vi "TAT_Varient Creater.vi"(8 "error in (no error)":errorcluster) -> (0 "error out":errorcluster)   [LabVIEW 2017]
uses:
  <vilib>/Utility/config.llb/Read Key (I32).vi
  <vilib>/Utility/config.llb/Write Key (U32).vi
  <vilib>/Utility/config.llb/NI_LVConfig.lvlib
  557cc533-a4ba-4953-a7b5-ba01b5e60265.vi
panel:
  in  "Cancle 2":bool
  in  "Delete Button":bool
  in  "Save Button":bool
  out "Varient Details":string[][](table)
  in  "SERIAL  NUMBER":u16=1 min=1 max=100 step=1
  in  "HOME":bool
  in  "UPDATE TABLE":bool
  in  "FG CAT No.":string(combo)
  # "Varient Creater"
  # "NOT IN USE"
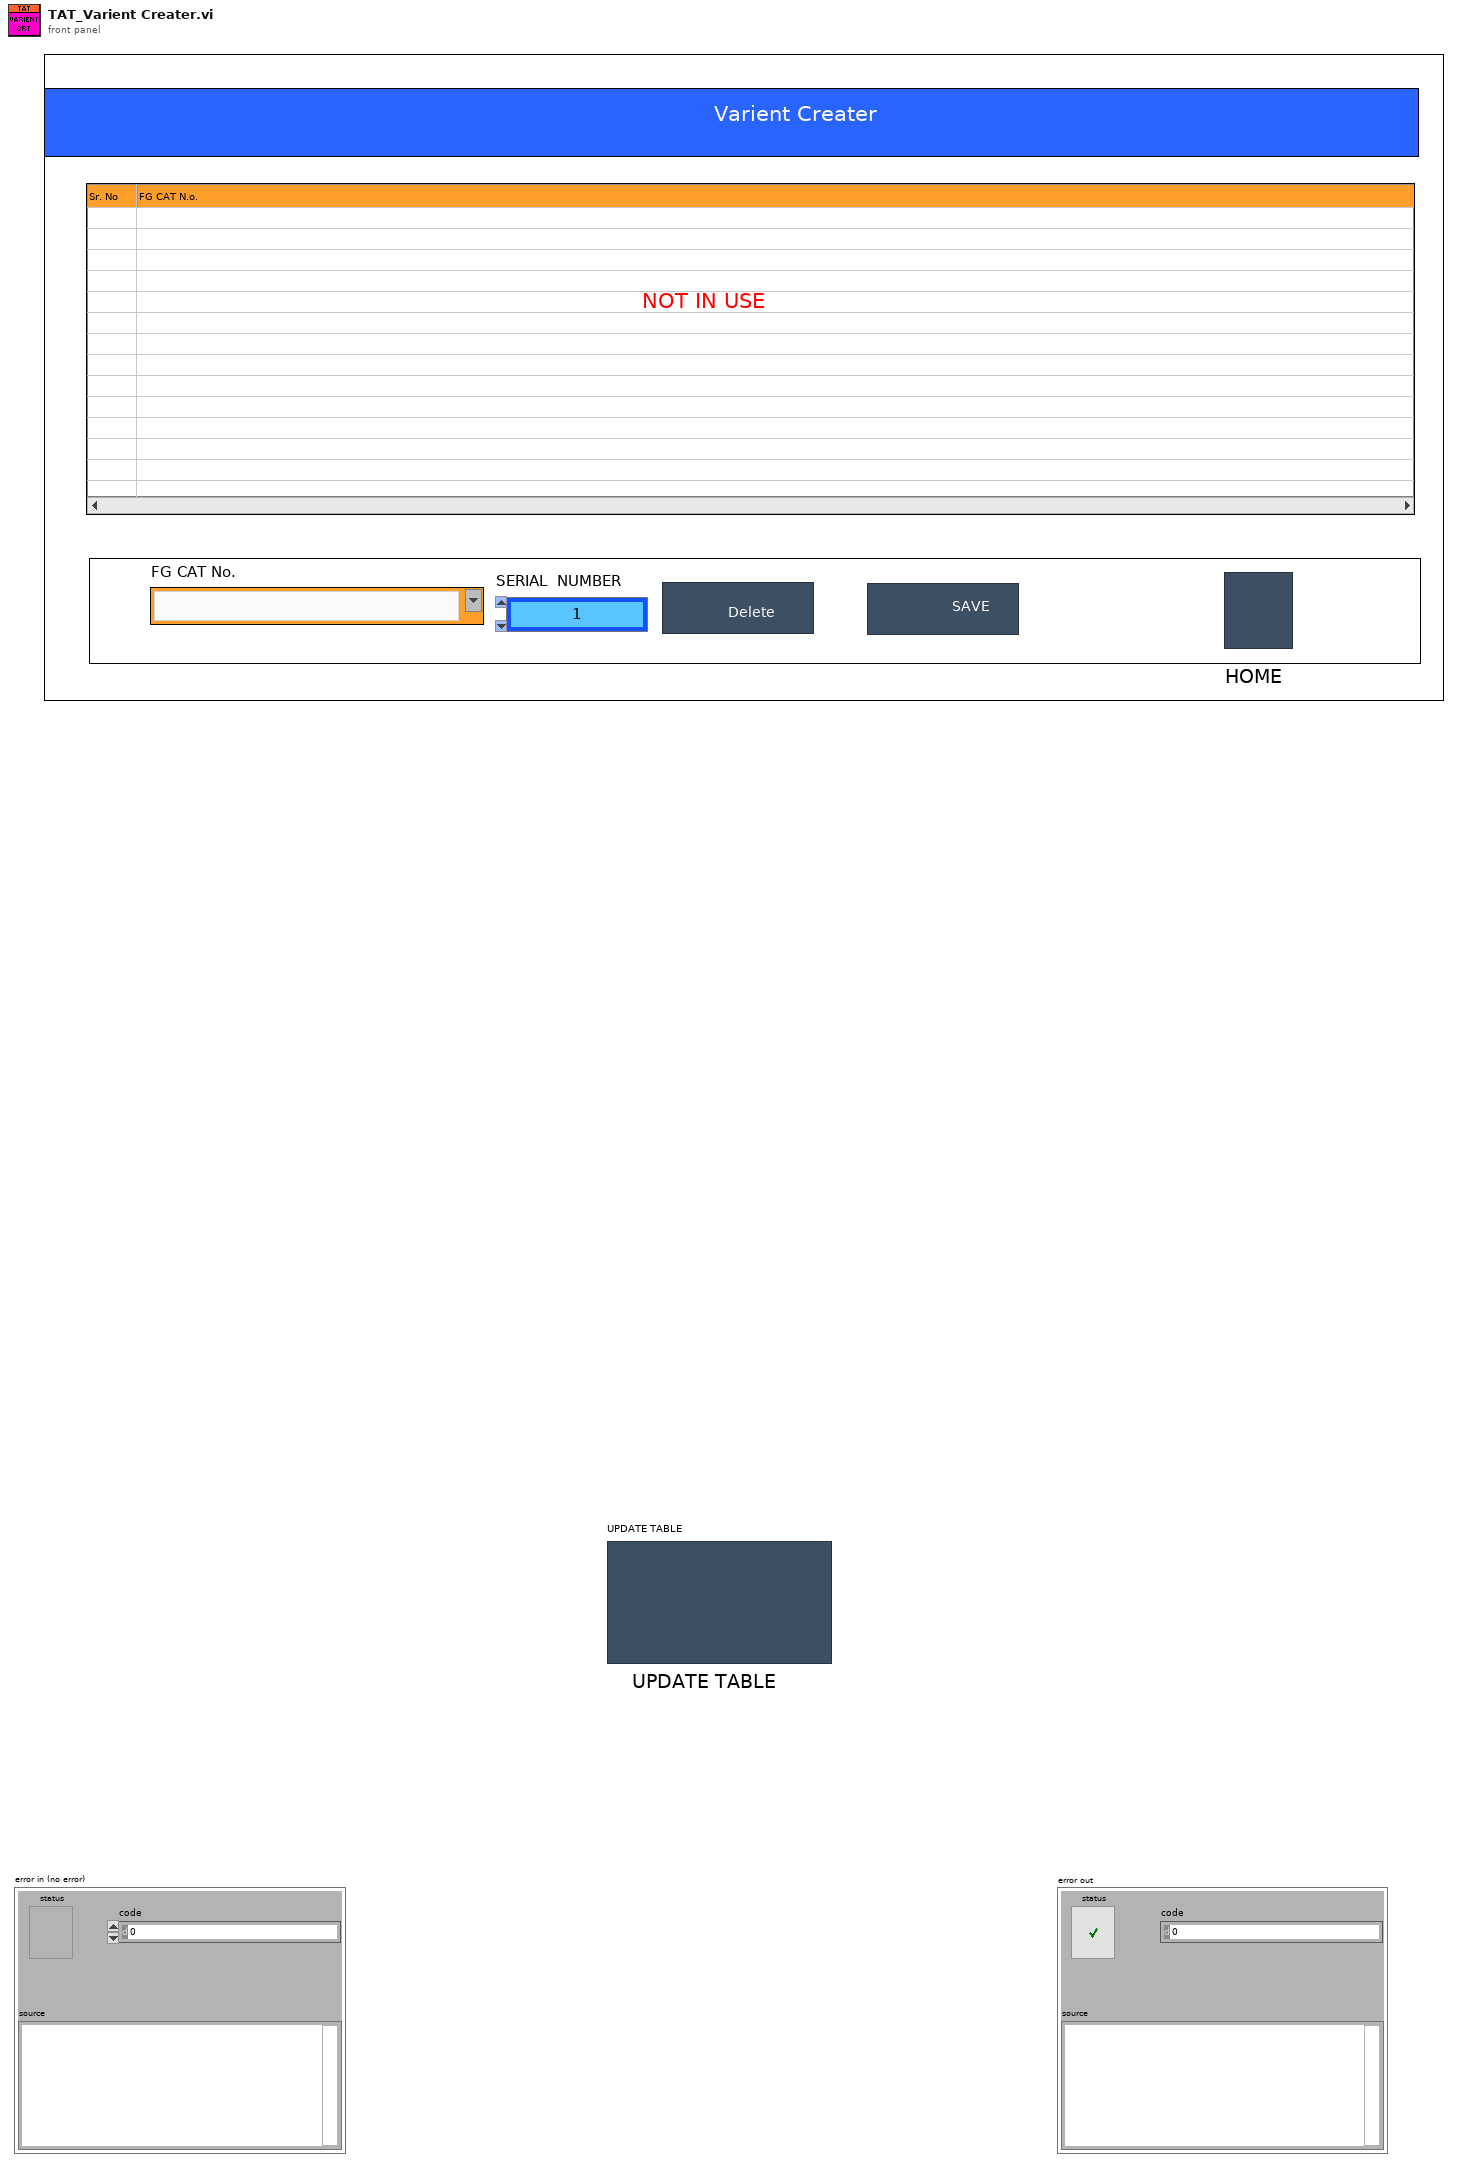
[diagram p1: front panel]
types:
  T1 = enum32{"invalid app kind", "Development System", "Run Time System", "Student Edition", "Embedded LabVIEW", "Evaluation", "Custom"}
  T2 = typedef "NI_LVConfig.lvlib/Config Data RefNum.ctl" = refnum<k1>
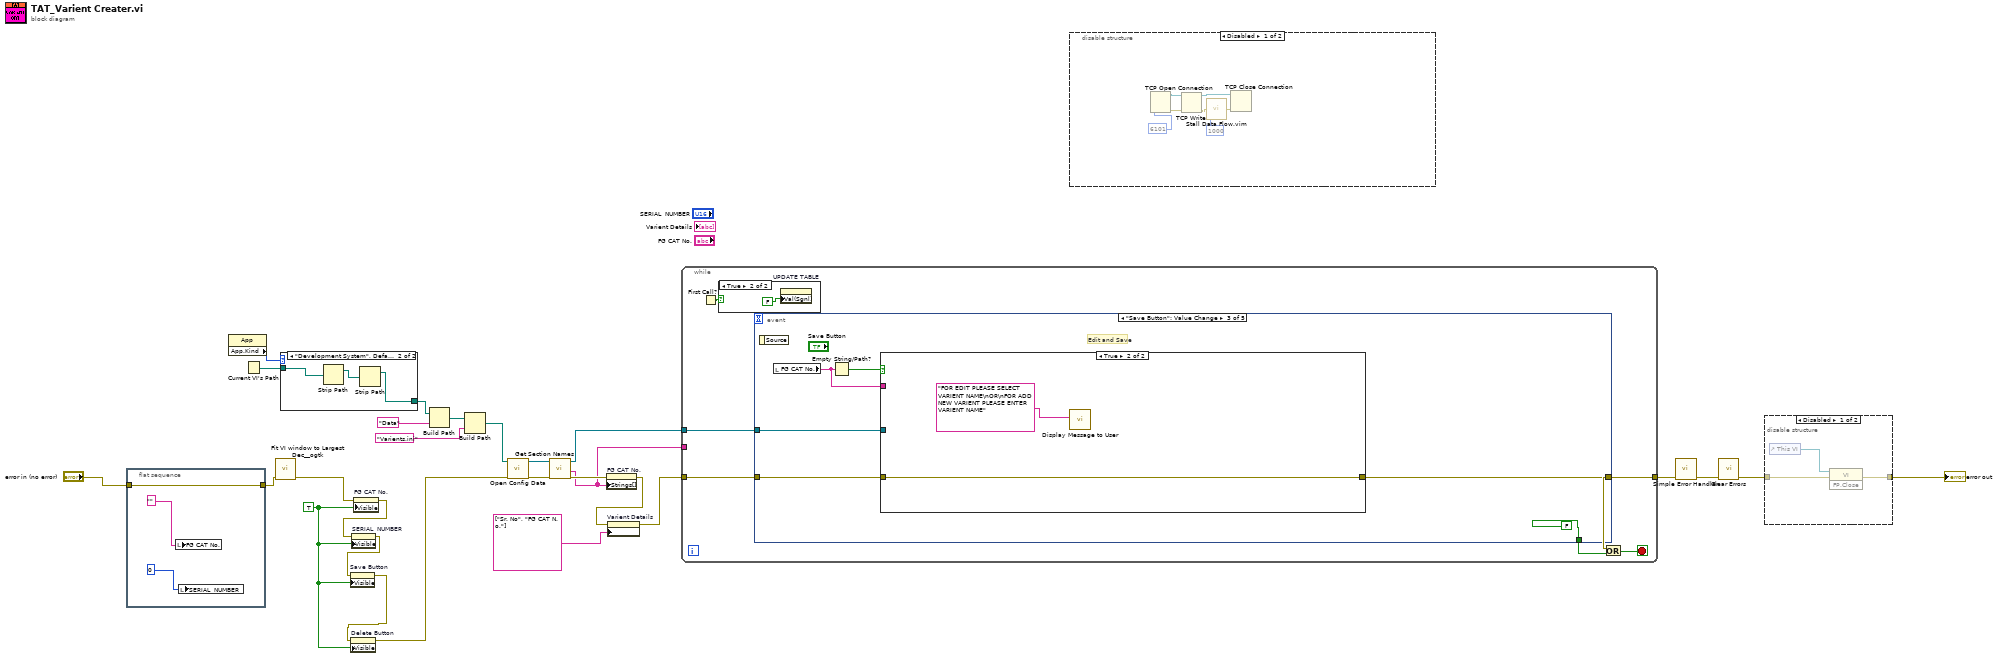
[diagram p0: block diagram]
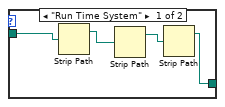
[diagram p4: hidden frame]
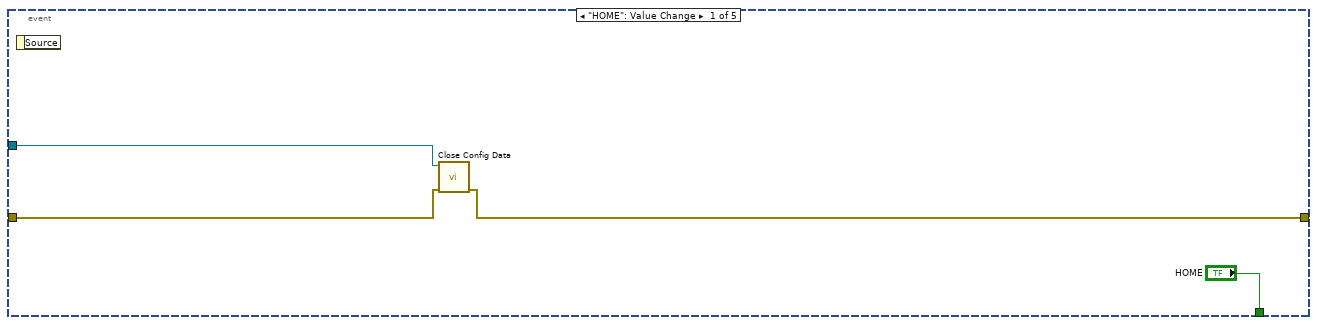
[diagram p6: hidden frame]
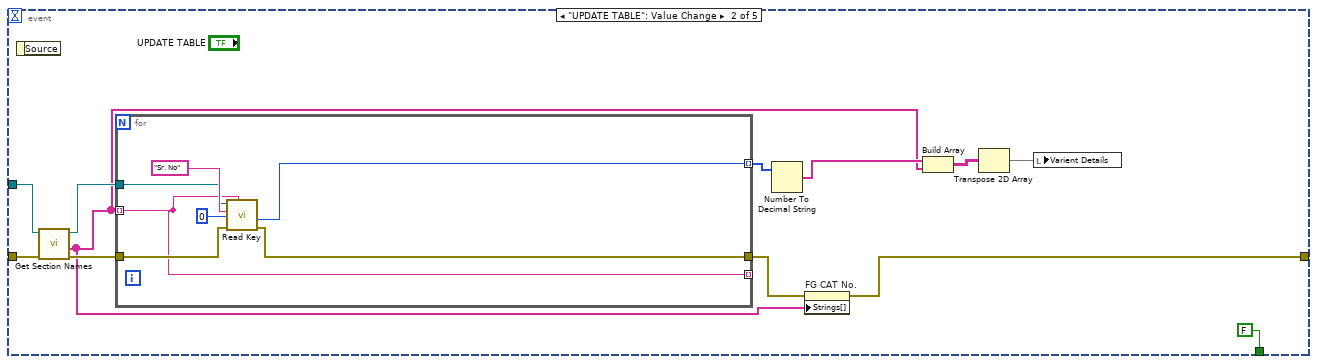
[diagram p7: hidden frame]
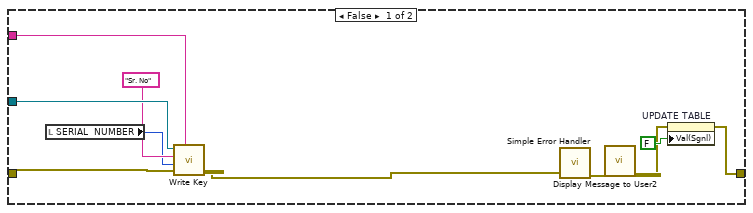
[diagram p8: hidden frame]
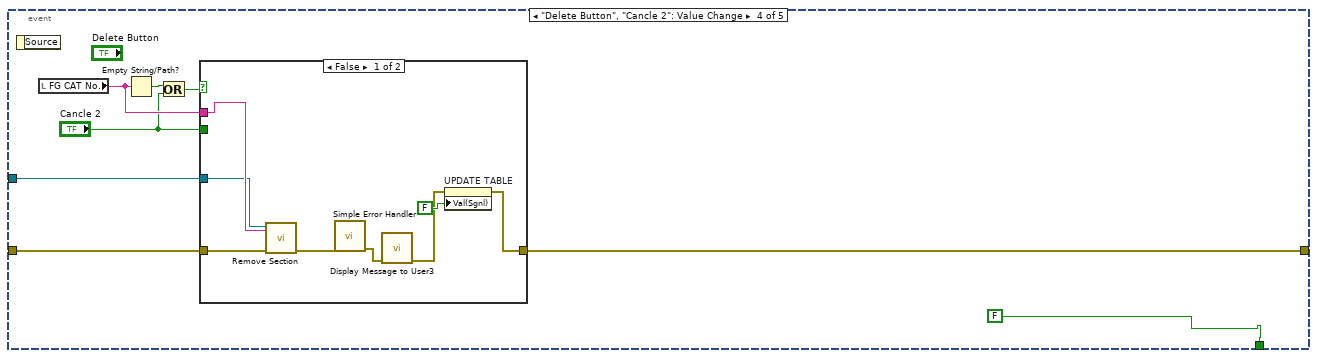
[diagram p9: hidden frame]
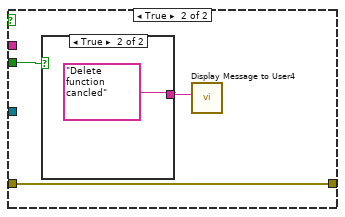
[diagram p10: hidden frame]
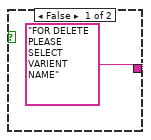
[diagram p11: hidden frame]
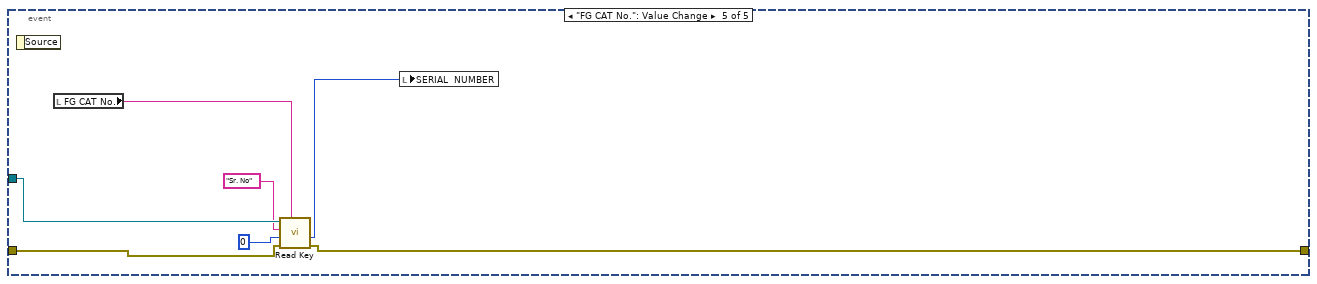
[diagram p12: hidden frame]
diagram:
  w5 = TRUE
  n1 = flat-sequence {
    tunnel: [w30] -> w10
    tunnel: "error in (no error)" -> [w30]
    frame #0 {
      n2 = local write "FG CAT No."("" ("PART NUMBER")) -> ()
      n3 = local write "SERIAL  NUMBER"(u16 0 ("BATCH SIZE")) -> ()
    }
  }
  n4 = property class="App"() -> ("App.Kind"=w22:T1)  [unwired: 2 in, 2 out]
  n5 = Current VI's Path() -> (path=w23:path)
  n6 = call <userlib>:"Fit VI window to Largest Dec__ogtk.vi"("error in (no error)"=w10) -> ("error out"=w3:errorcluster)  [unwired: 5 in, 1 out]
  n7 = case shown="\"Development System\", Default" w22 {
    tunnel: w23 -> [w32 w36]
    tunnel: [w31 w35] -> w6
    frame "Run Time System" {
      n8 = Strip Path(path=w32) -> (stripped path=w34:path)  [unwired: 1 out]
      n9 = Strip Path(path=w34) -> (stripped path=w33:path)  [unwired: 1 out]
      n10 = Strip Path(path=w33) -> (stripped path=w31:path)  [unwired: 1 out]
    }
    frame "Development System", Default {
      n11 = Strip Path(path=w36) -> (stripped path=w37:path)  [unwired: 1 out]
      n12 = Strip Path(path=w37) -> (stripped path=w35:path)  [unwired: 1 out]
    }
  }
  n13 = property on="FG CAT No." class="CmbBox"(error in=w3, "Visible"=w5) -> (error out=w9:errorcluster)  [unwired: 1 in, 1 out]
  n14 = property on="SERIAL  NUMBER" class="DigNum (strict)"(error in=w9, "Visible"=w5) -> (error out=w2:errorcluster)  [unwired: 1 in, 1 out]
  n15 = property on="Save Button" class="Bool"(error in=w2, "Visible"=w5) -> (error out=w1:errorcluster)  [unwired: 1 in, 1 out]
  n16 = property on="Delete Button" class="Bool"(error in=w1, "Visible"=w5) -> (error out=w8:errorcluster)  [unwired: 1 in, 1 out]
  n17 = Build Path(base path=w6, name or relative path="Data") -> (appended path=w7:path)
  n18 = Build Path(base path=w7, name or relative path="Varients.ini") -> (appended path=w21:path)
  n19 = call <vilib>:"Open Config Data.vi"("error in (no error)"=w8, "configuration file path"=w21) -> ("error out"=w17:errorcluster, "refnum"=w18:T2)  [unwired: 7 in, 1 out]
  n20 = call <vilib>:"Get Section Names.vi"("error in (no error)"=w17, "refnum"=w18) -> ("error out"=w16:errorcluster, "section names"=w12:string[], "refnum out"=w15:T2)  [unwired: 7 in]
  n21 = property on="FG CAT No." class="CmbBox"(error in=w16, "Strings[]"=w12) -> (error out=w14:errorcluster)  [unwired: 1 in, 1 out]
  n22 = property on="Varient Details" class="Tbl (strict)"(error in=w14, "Column Headers[]"=string[] ["Sr. No", "FG CAT N.o."]) -> (error out=w13:errorcluster)  [unwired: 1 in, 1 out]
  n23 = while {
    tunnel: w13 -> [w42]
    tunnel: [w40] -> w24
    tunnel: w15 -> [w39]
    tunnel: w12 -> [_]
    stop <- w41 stop-if-true
    n24 = First Call?() -> (First Call?: T/F=w38:bool)
    n25 = case shown="True" w38 {
      frame False {
      }
      frame True {
        n26 = property on="UPDATE TABLE" class="Bool (strict)"("Val(Sgnl)"=FALSE) -> ()  [unwired: 2 in, 2 out]
      }
    }
    n27 = event shown="[2] \"Save Button\": Value Change" {
      selector: _ -> [_ _ _ _ _]
      dyn-events: _ -> [_ _ _ _ _]
      timeout: _ -> [_ _ _ _ _]
      tunnel: ["HOME" FALSE ("stop") FALSE ("stop") FALSE ("stop") _] -> w43
      tunnel: w42 -> [w47 w56 w71 w91 w113]
      tunnel: [w46 w51 w69 w86 w108] -> w40
      tunnel: w39 -> [w45 w54 w72 w92 w112]
      event "HOME": Value Change {
        n28 = event-data() -> ()  [unwired: 1 in, 1 out]
        n29 = call <vilib>:"Close Config Data.vi"("error in (no error)"=w47, "refnum"=w45) -> ("error out"=w46:errorcluster)  [unwired: 8 in, 1 out]
      }
      event "UPDATE TABLE": Value Change {
        n30 = event-data() -> ()  [unwired: 1 in, 1 out]
        n31 = call <vilib>:"Get Section Names.vi"("error in (no error)"=w56, "refnum"=w54) -> ("error out"=w55:errorcluster, "section names"=w49:string[], "refnum out"=w53:T2)  [unwired: 7 in]
        n32 = for {
          tunnel: [w62] -> w52
          tunnel: w55 -> [w65]
          tunnel: w49 -> [w61] mode=indexing
          tunnel: w53 -> [w64]
          tunnel: [w63] -> w59 mode=indexing
          tunnel: [w61] -> _ mode=indexing
          n33 = call-poly <vilib>:"Read Key.vi"("section"=w61, "error in (no error)"=w65, "default value"=0, "key"="Sr. No", "refnum"=w64) -> ("error out"=w62:errorcluster, "value"=w63:i32)  [unwired: 3 in, 2 out]
        }
        n34 = Number To Decimal String(number=w59) -> (decimal integer string=w58:string[])  [unwired: 1 in]
        n35 = property on="FG CAT No." class="CmbBox"(error in=w52, "Strings[]"=w49) -> (error out=w51:errorcluster)  [unwired: 1 in, 1 out]
        n36 = Build Array(w58, w49) -> (w57:string[][])
        n37 = Transpose 2D Array(2D array=w57) -> (transposed array=w50:string[][])
        n38 = local write "Varient Details"(w50) -> ()
      }
      event "Save Button": Value Change {
        # "Edit and Save"
        n39 = event-data() -> ()  [unwired: 1 in, 1 out]
        n40 = local read "FG CAT No."() -> (w70:string)
        n41 = Empty String/Path?(string/path=w70) -> (empty?=w68:bool)
        n42 = case shown="True" w68 {
          tunnel: w71 -> [w83 w85]
          tunnel: [w79 w85] -> w69
          tunnel: w72 -> [w82 _]
          tunnel: w70 -> [w75 _]
          frame False {
            n43 = local read "SERIAL  NUMBER"() -> (w78:u16)
            n44 = call-poly <vilib>:"Write Key.vi"("section"=w75, "error in (no error)"=w83, "value"=w78, "key"="Sr. No", "refnum"=w82) -> ("error out"=w74:errorcluster)  [unwired: 4 in, 2 out]
            n45 = call <vilib>:"Simple Error Handler.vi"("error in (no error)"=w74) -> ("error out"=w77:errorcluster)  [unwired: 4 in, 4 out]
            n46 = call "Display Message to User2"("error in (no error)"=w77) -> ("error out"=w76:errorcluster)  [unwired: 9 in, 1 out]
            n47 = property on="UPDATE TABLE" class="Bool (strict)"(error in=w76, "Val(Sgnl)"=FALSE) -> (error out=w79:errorcluster)  [unwired: 1 in, 1 out]
          }
          frame True {
            n48 = call "Display Message to User"("Message"="FOR EDIT PLEASE SELECT VARIENT NAME\nOR\nFOR ADD NEW VARIENT PLEASE ENTER VARIENT NAME") -> ()  [unwired: 9 in, 2 out]
          }
        }
      }
      event "Delete Button", "Cancle 2": Value Change {
        n49 = event-data() -> ()  [unwired: 1 in, 1 out]
        n50 = local read "FG CAT No."() -> (w90:string)
        n51 = Empty String/Path?(string/path=w90) -> (empty?=w89:bool)
        n52 = Or(x=w89, y="Cancle 2") -> (x .or. y?=w88:bool)
        n53 = case shown="False" w88 {
          tunnel: w91 -> [w95 w104]
          tunnel: [w100 w104] -> w86
          tunnel: w92 -> [w96 _]
          tunnel: w90 -> [w97 _]
          tunnel: "Cancle 2" -> [_ w103]
          frame False {
            n54 = call <vilib>:"Remove Section.vi"("section"=w97, "error in (no error)"=w95, "refnum"=w96) -> ("error out"=w94:errorcluster)  [unwired: 6 in, 2 out]
            n55 = call <vilib>:"Simple Error Handler.vi"("error in (no error)"=w94) -> ("error out"=w99:errorcluster)  [unwired: 4 in, 4 out]
            n56 = call "Display Message to User3"("error in (no error)"=w99) -> ("error out"=w98:errorcluster)  [unwired: 9 in, 1 out]
            n57 = property on="UPDATE TABLE" class="Bool (strict)"(error in=w98, "Val(Sgnl)"=FALSE) -> (error out=w100:errorcluster)  [unwired: 1 in, 1 out]
          }
          frame True {
            n58 = case shown="True" w103 {
              tunnel: ["FOR DELETE PLEASE SELECT VARIENT NAME" "Delete function cancled"] -> w102
              frame False {
              }
              frame True {
              }
            }
            n59 = call "Display Message to User4"("Message"=w102) -> ()  [unwired: 9 in, 2 out]
          }
        }
      }
      event "FG CAT No.": Value Change {
        n60 = event-data() -> ()  [unwired: 1 in, 1 out]
        n61 = local read "FG CAT No."() -> (w107:string)
        n62 = call-poly <vilib>:"Read Key.vi"("section"=w107, "error in (no error)"=w113, "default value"=0, "key"="Sr. No", "refnum"=w112) -> ("error out"=w108:errorcluster, "value"=w110:i32)  [unwired: 3 in, 2 out]
        n63 = local write "SERIAL  NUMBER"(w110) -> ()
      }
    }
    n64 = Or(x=w40, y=w43) -> (x .or. y?=w41:bool)
  }
  n65 = disable-structure shown="Disabled" {
    frame Disabled {
      n66 = TCP Open Connection(remote port or service name=u16 6101) -> (connection ID=w119:refnum<k5>, error out=w118:errorcluster)  [unwired: 4 in]
      n67 = TCP Write(connection ID=w119, error in (no error)=w118) -> (connection ID out=w121:refnum<k5>, error out=w117:errorcluster)  [unwired: 2 in, 1 out]
      n68 = call "Stall Data Flow.vim"("value in"=w117, "milliseconds to wait"=u32 1000) -> ("value out"=w120:errorcluster)  [unwired: 1 out]
      n69 = TCP Close Connection(connection ID=w121, error in (no error)=w120) -> (error out=w114:errorcluster)  [unwired: 1 in, 1 out]
    }
    frame Enabled {
    }
  }
  n70 = call <vilib>:"Simple Error Handler.vi"("error in (no error)"=w24) -> ("error out"=w27:errorcluster)  [unwired: 4 in, 4 out]
  n71 = call <vilib>:"Clear Errors.vi"("error in (no error)"=w27) -> ("error out"=w26:errorcluster)  [unwired: 5 in, 1 out]
  n72 = disable-structure shown="Disabled" {
    disable-tunnel: w26 -> [w124 w125]
    disable-tunnel: [w123 w125] -> w25
    frame Disabled {
      n73 = control-ref of="This VI"() -> (w122:refnum<vi>)
      n74 = invoke class="VI" method="FP.Close"(reference=w122, error in=w124) -> (error out=w123:errorcluster)  [unwired: 1 in, 2 out]
    }
    frame Enabled {
    }
  }
  "error out" <- w25
